vi "From JSON.vi"(8 "error in (no error)":errorcluster, 10 "JSON":string, 11 "Type in":refnum<class "Abs_Boolean_1D.lvclass">) -> (0 "error out":errorcluster, 3 "Type out":refnum<class "Abs_Boolean_1D.lvclass">)   [LabVIEW 2021, in "Abs_Boolean_1D.lvclass"]
uses:
  Abs_Boolean_1D.lvclass
  C:/Program Files (x86)/National Instruments/LabVIEW 2021/vi.lib/TSA/Abstract Data Classes/Abs_Types/Type/Abs_Type.lvclass
  Support/Element Type.ctl
  ef96c86a-dc6b-4f38-b092-0a6ef853fecf.vi
  <vilib>/JDP Science/JSONtext/Find Item.vi
  <vilib>/JDP Science/JSONtext/Next JSON Value.vi
  <vilib>/JDP Science/JSONtext/String Subset.vi
  <vilib>/JDP Science/JSONtext/Parsing/Advance past next JSON Value (inlined COPY).vi
  <vilib>/JDP Science/JSONtext/Parsing/Advance past whitespace.vi
  <vilib>/JDP Science/JSONtext/Parsing/Advance past String.vi
  <vilib>/JDP Science/JSONtext/Parsing/Advance past Number.vi
  <vilib>/JDP Science/JSONtext/Parsing/Advance past Line Ending.vi
  <vilib>/Utility/LVClass/Get LV Class Name.vi
  <vilib>/JDP Science/JSONtext/Parsing/Parse Full Path or Item Name.vi
  <vilib>/JDP Science/JSONtext/Parsing/Advance past Array.vi
  <vilib>/JDP Science/JSONtext/Parsing/Advance past Object.vi
  <vilib>/JDP Science/JSONtext/support/Error Cluster From Code.vi
  <vilib>/JDP Science/JSONtext/Offset/Find Item Locations by Path.vi
  <vilib>/JDP Science/JSONtext/JSON text to Variant.vi
  <vilib>/JDP Science/JSONtext/LVClass Serializer/JSONtext LVClass Serializer.lvclass
  Array 1D/Abs_Array1D.lvclass
  Type/Abs_Type.lvclass
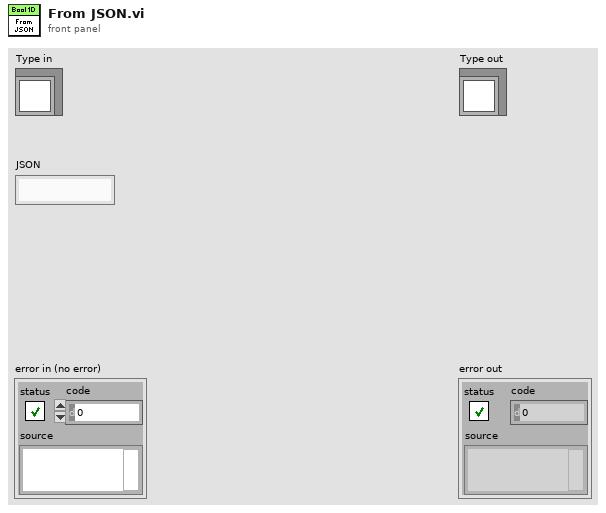
[diagram p1: front panel]
types:
  T1 = typedef "Abs_Boolean_1D.lvclass/Element Type.ctl" = bool
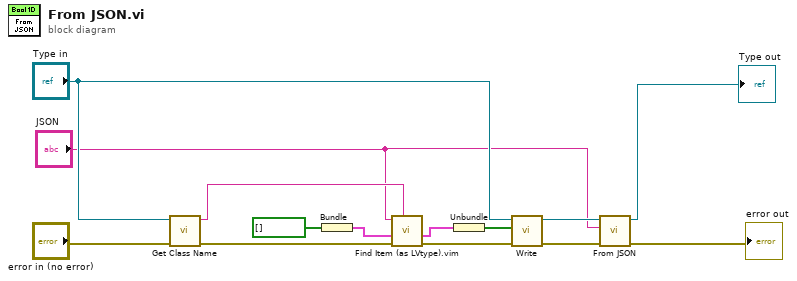
[diagram p0: block diagram]
diagram:
  n1 = call "Get Class Name.vi"("error in (no error)"="error in (no error)", "Abs_Type in"="Type in") -> ("error out"=w11:errorcluster, "class name"=w12:string)  [unwired: 8 in]
  n2 = Bundle("Boolean 1D"=T1[] []) -> (w13:cluster{"Boolean 1D":T1[]})  [unwired: 1 in]
  n3 = call "Find Item (as LVtype).vim"("$Path or Item Name"=w12, "error in (no error)"=w11, "Data Type and Default Value"=w13, "JSON"="JSON") -> ("error out"=w10:errorcluster, "Data"=w14:cluster{"Boolean 1D":T1[]})  [unwired: 4 in, 2 out]
  n4 = Unbundle(w14) -> ("Boolean 1D"=w7:T1[])
  n5 = call-dynamic "Write.vi"("error in (no error)"=w10, "Boolean 1D"=w7, "Boolean in"="Type in") -> ("error out"=w9:errorcluster, "Boolean out"=w8:refnum<class "Abs_Boolean_1D.lvclass">)  [unwired: 7 in]
  n6 = call-parent "From JSON.vi"("error in (no error)"=w9, "JSON"="JSON", "Type in"=w8) -> ("error out"=→"error out":errorcluster, "Type out"=→"Type out":refnum<class "Abs_Boolean_1D.lvclass">)  [unwired: 7 in]
